vi "Determine Clicked Array Element Index - Test For Error Code 1320.vi"(7 "error in":errorcluster) -> (8 "error out":errorcluster)   [LabVIEW 2011]
doc: "Determine Clicked Array Element Index - Test For Error Code 1320.vi\n\nDescription:\nThis VI determines determines if error code 1320 has occured, and if so, instructs the user how to correct the issue and cancels the error.\n\nInputs:\nerror in - Standard error cluster.\n\nOutputs:\nerror out - standard error cluster.\n\nDeveloped By:\nMark.ridgley\nMark.Ridgley_LabVIEW.Developer@comcast.net"
panel:
  # "Error 1320 indicates that in run mode, LabVIEW cannot get or set a property for a control part that has not been created. Arrays drop with the caption undefined, so we need to instruct the user how to correct this issue."
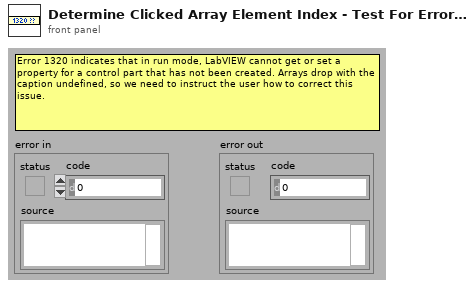
[diagram p1: front panel]
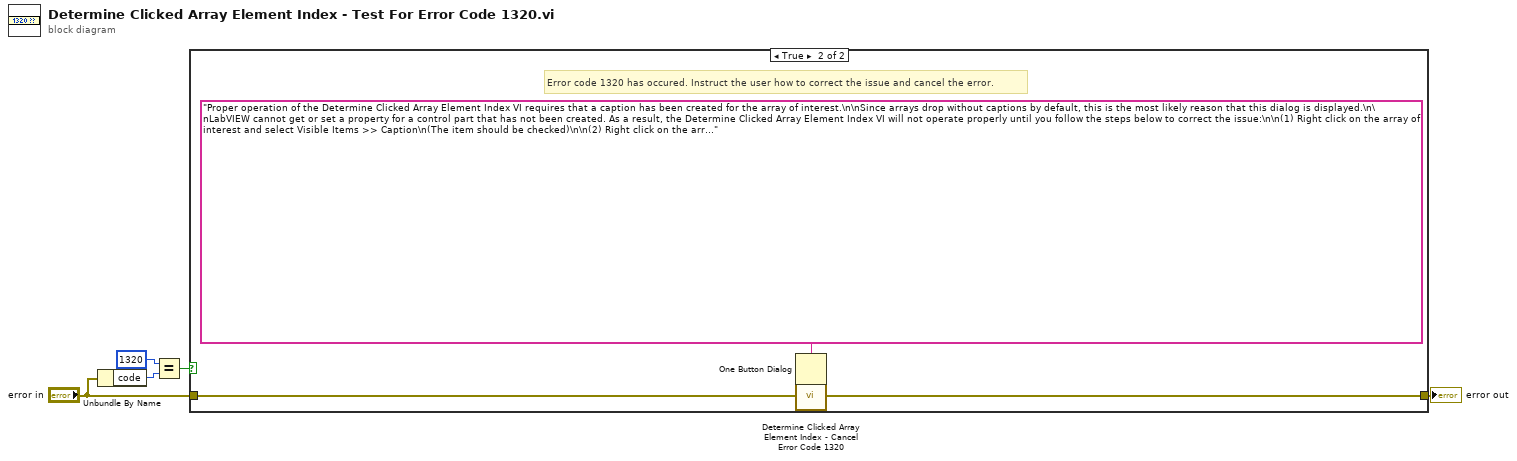
[diagram p0: block diagram]
diagram:
  n1 = Unbundle By Name("error in") -> ("code"=w5:i32)
  n2 = Equal?(x=1320 ("[exception code]"), y=w5) -> (x = y?=w3:bool)
  n3 = case shown="True" w3 {
    tunnel: "error in" -> [w6 w9]
    tunnel: [w6 w8] -> w1
    frame False {
    }
    frame True {
      # "Error code 1320 has occured. Instruct the user how to correct the issue and cancel the error."
      n4 = One Button Dialog(message="Proper operation of the Determine Clicked Array Element Index VI requires that a caption has been created for the array of interest.\n\nSince arrays drop without captions by default, this is the most likely reason that this dialog is displayed.\n\nLabVIEW cannot get or set a property for a control part that has not been created. As a result, the Determine Clicked Array Element Index VI will not operate properly until you follow the steps below to correct the issue:\n\n(1) Right click on the array of interest and select Visible Items >> Caption\n(The item should be checked)\n\n(2) Right click on the array of interest and select Visible Items >> Caption\n(The item should be un-checked)\n\n(3) Right click on the array of interest and select Visible Items >> Label\n(The item should be checked)\n\n(4) Save the VI") -> ()  [unwired: 1 in, 1 out]
      n5 = call "Determine Clicked Array Element Index - Cancel Error Code 1320.vi"("error in"=w9) -> ("error out"=w8:errorcluster)  [unwired: 14 in]
    }
  }
  "error out" <- w1
